vi "Init.vi"(6 "Signal Suffix":string, 8 "error in (no error)":errorcluster, 9 "SA Pin":string, 10 "Measurement Name":string, 11 "Standard":string) -> (0 "error out":errorcluster, 3 "IMD_ACP out":refnum<class "IMD_ACP.lvclass">)   [LabVIEW 2018, in "SeqAuto Evaluations.lvlib" / "IMD_ACP.lvclass"]
uses:
  IMD_ACP.lvclass
  C:/Sequence Automation/Plugins/SeqAuto IEvaluation.lvlibp/SeqAuto IEvaluation.lvclass
  IMD_ACP.lvclass/IMD_ACP.ctl
  Write Signal Suffix.vi
  Write SA Pin.vi
  Plugins/SeqAuto IEvaluation.lvlibp/Write Measurement Name.vi
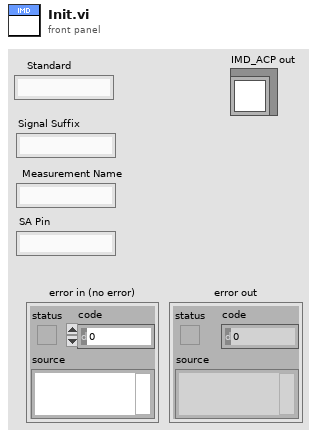
[diagram p1: front panel]
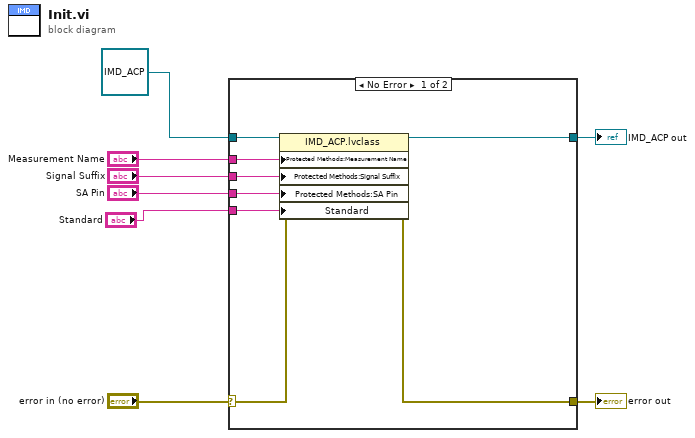
[diagram p0: block diagram]
diagram:
  n1 = case shown="No Error" "error in (no error)" {
    selector: "error in (no error)" -> [w16 w18]
    tunnel: [w15 w18] -> w7
    tunnel: refnum<class "IMD_ACP.lvclass"> refnum ("IMD_ACP in") -> [w14 w17]
    tunnel: "Measurement Name" -> [w13 _]
    tunnel: "SA Pin" -> [w12 _]
    tunnel: "Signal Suffix" -> [w11 _]
    tunnel: [w10 w17] -> w3
    tunnel: "Standard" -> [w9 _]
    frame No Error {
      n2 = property class="IMD_ACP.lvclass"(reference=w14, error in=w16, "Protected Methods:Measurement Name"=w13, "Protected Methods:Signal Suffix"=w11, "Protected Methods:SA Pin"=w12, "Standard"=w9) -> (reference out=w10:refnum<class "IMD_ACP.lvclass">, error out=w15:errorcluster)
    }
    frame Error {
    }
  }
  "error out" <- w7
  "IMD_ACP out" <- w3
